vi "Read Size.vi"(8 "error in (no error)":errorcluster, 11 "Sequence in":refnum<class "Sequence.lvclass">) -> (0 "error out":errorcluster, 2 "Size":i32, 3 "Sequence out":refnum<class "Sequence.lvclass">)   [LabVIEW 2015, in "Sequence.lvclass"]
uses:
  Sequence.lvclass
  Sequence.lvclass/Sequence.ctl
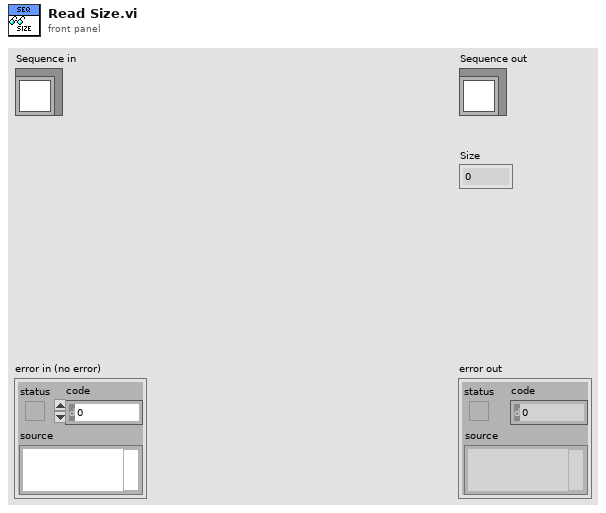
[diagram p1: front panel]
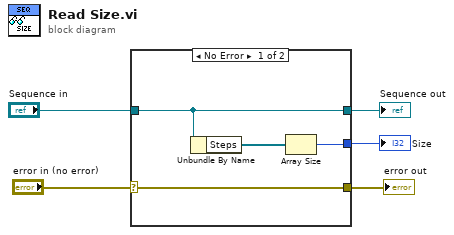
[diagram p0: block diagram]
diagram:
  n1 = case shown="No Error" "error in (no error)" {
    selector: "error in (no error)" -> [w9 w11]
    tunnel: [w9 w11] -> w4
    tunnel: [w8 w10] -> w2
    tunnel: "Sequence in" -> [w8 w10]
    tunnel: [w6 _] -> w1
    frame No Error {
      n2 = Unbundle By Name(w8) -> ("Steps"=w7:refnum<class "Step.lvclass">[])
      n3 = Array Size(array=w7) -> (size(s)=w6:i32)
    }
    frame Error {
    }
  }
  "error out" <- w4
  "Sequence out" <- w2
  "Size" <- w1
